vi "Meacurrent8341.vi"(10 "测试类型":u16(ring) items=["DCV", "ACV", "DCI", "ACI", "OHM", "RST", "CAP", "FRQ", "AUTO"], 11 "VISA资源名称":refnum<visa-resource-name>="COM1") -> (0 "错误输出":errorcluster, 2 "数值":dbl format="%#_3g")   [LabVIEW 2013]
uses:
  C:/Program Files/National Instruments/LabVIEW 2013/examples/Instrument IO/Serial/support/Serial - Settings.ctl
  <vilib>/Instr/_visa.llb/VISA Flush IO Buffer Mask.ctl
  <vilib>/Instr/_visa.llb/VISA Configure Serial Port (Instr).vi
panel:
  out "响应":string
  in  "串口设置":T1={"波特率"=9600, "数据比特"=8, "奇偶"=enum."None", "停止位"=10, "流控制"=0} {"流控制" items=["无"=0, "XON/XOFF"=1, "RTS/CTS"=2, "DTR/DSR"=4]; "停止位" items=["1.0"=10, "1.5"=15, "2.0"=20]; "数据比特" min=5 max=8 step=1; "波特率" items=["75"=75, "110"=110, "134"=134, "150"=150, "300"=300, "600"=600, "1200"=1200, "1800"=1800, "2400"=2400, "4800"=4800, "7200"=7200, "9600"=9600, "14400"=14400, "19200"=19200, "28800"=28800, "38400"=38400, "56000"=56000, "57600"=57600, "115200"=115200, "128000"=128000, "230400"=230400]}
  in  "读取前延时(ms)":u32=600
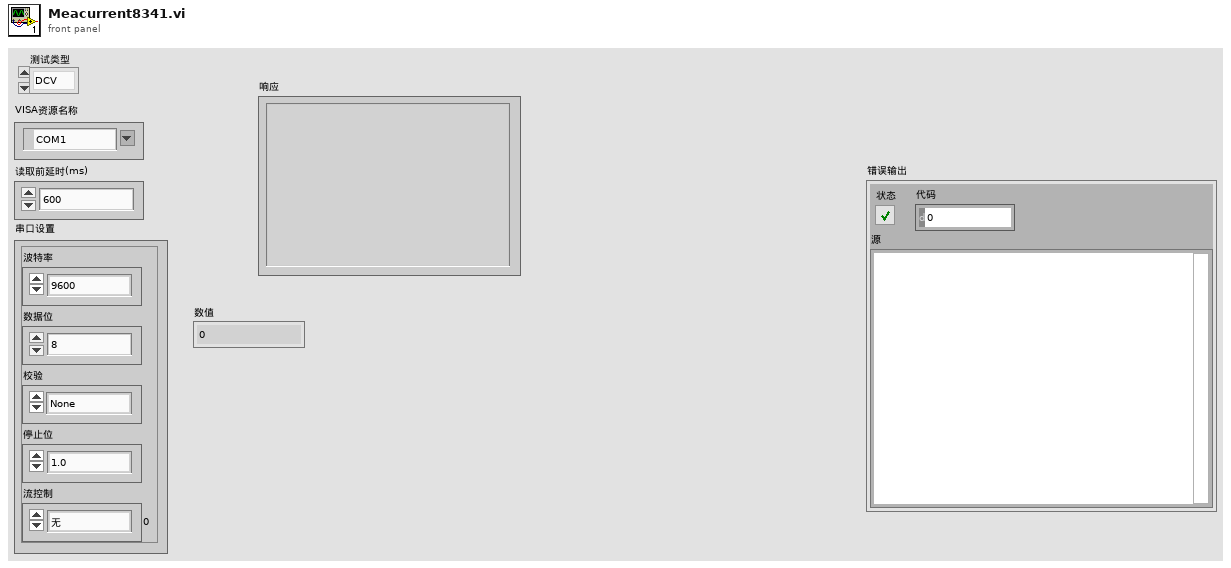
[diagram p1: front panel]
types:
  T1 = typedef "Serial - Settings.ctl" = cluster{"波特率":u32, "数据比特":u16, "奇偶":enum16{"None", "Odd", "Even", "Mark", "Space"}, "停止位":u16, "流控制":u16}
  T2 = typedef "VISA Flush IO Buffer Mask.ctl" = u16
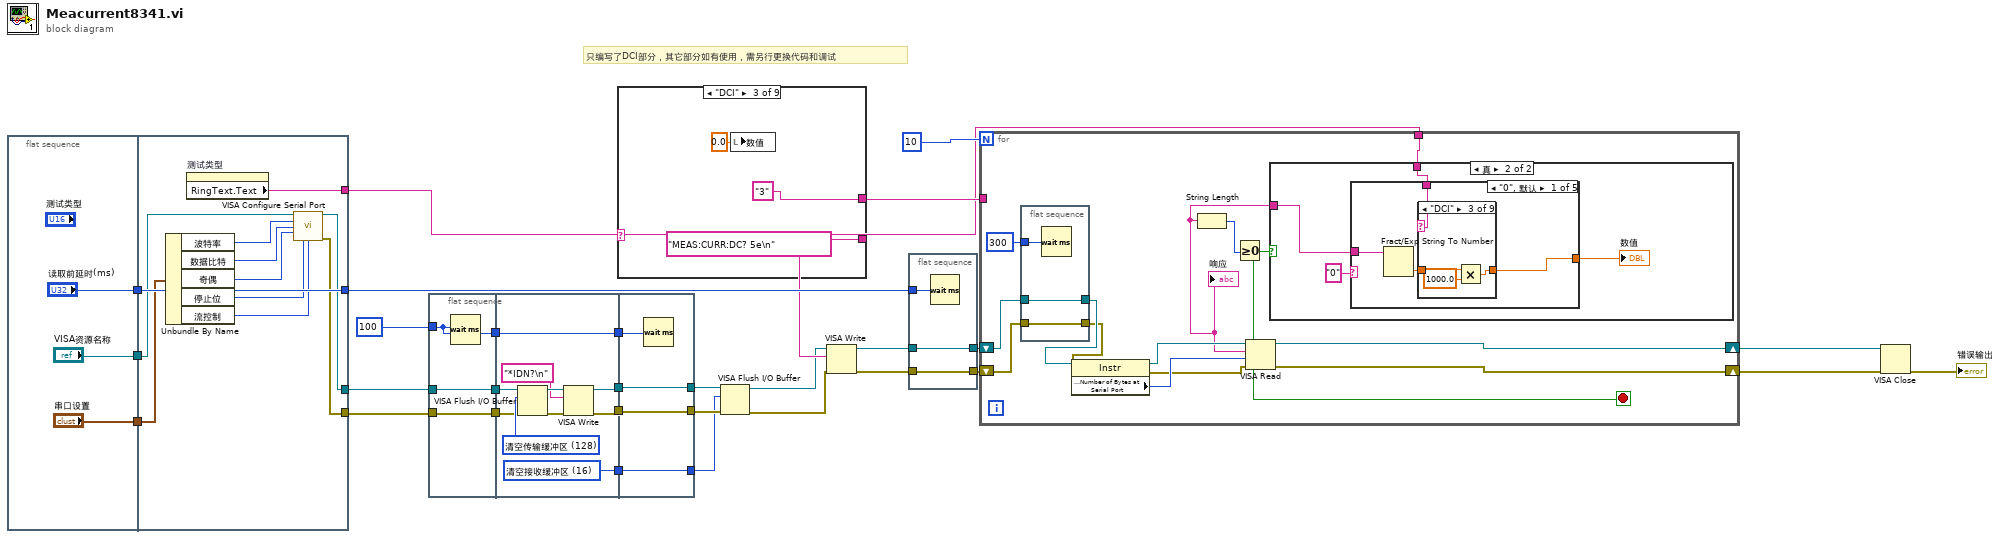
[diagram p0: block diagram]
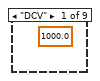
[diagram p3: hidden frame]
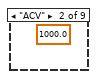
[diagram p4: hidden frame]
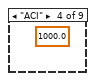
[diagram p5: hidden frame]
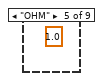
[diagram p6: hidden frame]
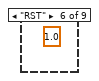
[diagram p7: hidden frame]
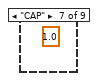
[diagram p8: hidden frame]
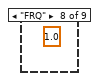
[diagram p9: hidden frame]
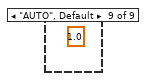
[diagram p10: hidden frame]
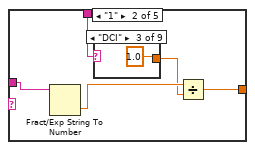
[diagram p11: hidden frame]
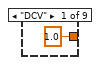
[diagram p12: hidden frame]
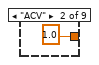
[diagram p13: hidden frame]
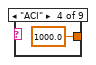
[diagram p14: hidden frame]
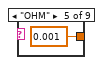
[diagram p15: hidden frame]
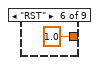
[diagram p16: hidden frame]
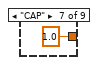
[diagram p17: hidden frame]
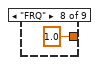
[diagram p18: hidden frame]
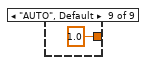
[diagram p19: hidden frame]
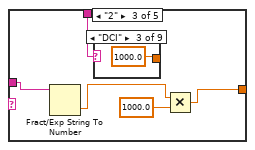
[diagram p20: hidden frame]
diagram:
  # "只编写了DCI部分，其它部分如有使用，需另行更换代码和调试"
  n1 = flat-sequence {
    tunnel: ["VISA资源名称"] -> w8
    tunnel: ["读取前延时(ms)"] -> w7
    tunnel: ["串口设置"] -> w6
    tunnel: [w44] -> w26
    tunnel: w8 -> [w37]
    tunnel: w7 -> [w44]
    tunnel: w6 -> [w38]
    tunnel: [w36] -> w4
    tunnel: [w35] -> w2
    tunnel: [w34] -> w1
    frame #0 {
    }
    frame #1 {
      n2 = Unbundle By Name(w38) -> ("波特率"=w39:u32, "数据比特"=w40:u16, "奇偶"=w41:enum16{"None", "Odd", "Even", "Mark", "Space"}, "停止位"=w42:u16, "流控制"=w43:u16)
      n3 = property on="测试类型" class="Ring (严格)"() -> ("RingText.Text"=w34:string)  [unwired: 2 in, 2 out]
      n4 = call-poly "VISA Configure Serial Port"("VISA resource name"=w37, "baud rate (9600)"=w39, "data bits (8)"=w40, "parity (0:none)"=w41, "stop bits (10: 1 bit)"=w42, "flow control (0:none)"=w43) -> ("VISA resource name out"=w36:refnum<visa-resource-name>, "error out"=w35:errorcluster)  [unwired: 3 in, 5 out]
    }
  }
  n5 = flat-sequence {
    tunnel: u32 100 ("读取前延时(ms)") -> [w47]
    tunnel: [w47] -> w17
    tunnel: [w46] -> w5
    tunnel: w4 -> [w46]
    tunnel: [w45] -> w3
    tunnel: w2 -> [w45]
    tunnel: [w52] -> w20
    tunnel: [w53] -> w19
    tunnel: [w51] -> w18
    tunnel: w17 -> [w51]
    tunnel: [w50] -> w16
    tunnel: w5 -> [w49]
    tunnel: w3 -> [w48]
    tunnel: [w59] -> w13
    tunnel: [w60] -> w12
    tunnel: w20 -> [w60]
    tunnel: w19 -> [w59]
    tunnel: w18 -> [w61]
    tunnel: w16 -> [w58]
    tunnel: [w58] -> w11
    frame #0 {
      n6 = Wait (ms)(milliseconds to wait=w47) -> ()  [unwired: 1 out]
    }
    frame #1 {
      w50 = T2 16 items=["清空接收缓冲区"=16, "向设备写入传输缓冲区"=32, "清空接收缓冲区（无I/O）"=64, "清空传输缓冲区"=128] ("Mask")
      w57 = T2 128 items=["清空接收缓冲区"=16, "向设备写入传输缓冲区"=32, "清空接收缓冲区（无I/O）"=64, "清空传输缓冲区"=128] ("Mask")
      n7 = VISA Flush I/O Buffer(VISA resource name=w49, mask (16)=w57, error in (no error)=w48) -> (VISA resource name out=w55:refnum<visa-resource-name>, error out=w56:errorcluster)
      n8 = VISA Write(VISA resource name=w55, write buffer="*IDN?\n" ("写入缓冲区"), error in (no error)=w56) -> (VISA resource name out=w53:refnum<visa-resource-name>, error out=w52:errorcluster)  [unwired: 1 out]
    }
    frame #2 {
      n9 = Wait (ms)(milliseconds to wait=w61) -> ()  [unwired: 1 out]
    }
  }
  n10 = case shown="\"DCI\"" w1 {
    tunnel: ["AA" ("Command") "BB" ("Command") "MEAS:CURR:DC? 5e\n" "DD" ("Command") "EE" ("Command") "FF" ("Command") "GG" ("Command") "HH" ("Command") "MM" ("Command")] -> w25
    tunnel: ["0" ("Command") "1" ("Command") "3" ("Command") "4" ("Command") "6" ("Command") "F" ("Command") "7" ("Command") "8" ("Command") "M" ("Command")] -> w24
    frame "DCV" {
    }
    frame "ACV" {
    }
    frame "DCI" {
      n11 = local write "数值"(0.0 ("数值")) -> ()
    }
    frame "ACI" {
    }
    frame "OHM" {
    }
    frame "RST" {
    }
    frame "CAP" {
    }
    frame "FRQ" {
    }
    frame "AUTO", Default {
    }
  }
  n12 = VISA Flush I/O Buffer(VISA resource name=w13, mask (16)=w11, error in (no error)=w12) -> (VISA resource name out=w9:refnum<visa-resource-name>, error out=w10:errorcluster)
  n13 = VISA Write(VISA resource name=w9, write buffer=w25, error in (no error)=w10) -> (VISA resource name out=w15:refnum<visa-resource-name>, error out=w14:errorcluster)  [unwired: 1 out]
  n14 = flat-sequence {
    tunnel: [w81] -> w28
    tunnel: [w82] -> w27
    tunnel: w26 -> [w83]
    tunnel: w15 -> [w82]
    tunnel: w14 -> [w81]
    frame #0 {
      n15 = Wait (ms)(milliseconds to wait=w83) -> ()  [unwired: 1 out]
    }
  }
  n16 = for {
    N: 10 -> [_]
    tunnel: w24 -> [_]
    tunnel: w1 -> [w94]
    shift-right: [w96] -> w29
    shift-left: w27 -> [w93]
    shift-right: [w97] -> w30
    shift-left: w28 -> [w91]
    stop <- w88 stop-if-true
    n17 = flat-sequence {
      tunnel: w91 -> [w99]
      tunnel: [w99] -> w90
      tunnel: w93 -> [w98]
      tunnel: [w98] -> w92
      tunnel: u32 300 ("读取前延时(ms)") -> [w100]
      frame #0 {
        n18 = Wait (ms)(milliseconds to wait=w100) -> ()  [unwired: 1 out]
      }
    }
    n19 = property class="Instr"(reference=w92, error in=w90) -> (reference out=w87:refnum<visa-resource-name>, error out=w86:errorcluster, "Serial Settings:Number of Bytes at Serial Port"=w95:u32)
    n20 = VISA Read(VISA resource name=w87, byte count=w95, error in (no error)=w86) -> (VISA resource name out=w96:refnum<visa-resource-name>, read buffer=w84:string, error out=w97:errorcluster)  [unwired: 1 out]
    "响应" <- w84
    n21 = String Length(string=w84) -> (length=w85:i32)
    n22 = Greater Or Equal To 0?(x=w85) -> (x >= 0?=w88:bool)
    n23 = case shown="真" w88 {
      tunnel: w84 -> [_ w101]
      tunnel: w94 -> [_ w104]
      frame False {
      }
      frame True {
        n24 = case shown="\"0\", 默认" "0" {
          tunnel: w101 -> [w108 w116 w130 w144 w158]
          tunnel: w104 -> [w107 w115 w129 w143 w157]
          tunnel: [w106 w112 w126 w140 w154] -> w103
          frame "0", Default {
            n25 = Fract/Exp String To Number(string=w108) -> (number=w105:dbl)  [unwired: 3 in, 1 out]
            n26 = case shown="\"DCI\"" w107 {
              tunnel: [_ _ w109 _ _ _ _ _ _] -> w106
              tunnel: w105 -> [_ _ w111 _ _ _ _ _ _]
              frame "DCV" {
                (unwired) 1000.0
              }
              frame "ACV" {
                (unwired) 1000.0
              }
              frame "DCI" {
                n27 = Multiply(x=w111, y=1000.0) -> (x*y=w109:dbl)
              }
              frame "ACI" {
                (unwired) 1000.0
              }
              frame "OHM" {
                (unwired) 1.0
              }
              frame "RST" {
                (unwired) 1.0
              }
              frame "CAP" {
                (unwired) 1.0
              }
              frame "FRQ" {
                (unwired) 1.0
              }
              frame "AUTO", Default {
                (unwired) 1.0
              }
            }
          }
          frame "1" {
            n28 = Fract/Exp String To Number(string=w116) -> (number=w114:dbl)  [unwired: 3 in, 1 out]
            n29 = case shown="\"DCI\"" w115 {
              tunnel: [1.0 1.0 1.0 1000.0 0.001 1.0 1.0 1.0 1.0] -> w113
              frame "DCV" {
              }
              frame "ACV" {
              }
              frame "DCI" {
              }
              frame "ACI" {
              }
              frame "OHM" {
              }
              frame "RST" {
              }
              frame "CAP" {
              }
              frame "FRQ" {
              }
              frame "AUTO", Default {
              }
            }
            n30 = Divide(x=w114, y=w113) -> (x/y=w112:dbl)
          }
          frame "2" {
            n31 = Fract/Exp String To Number(string=w130) -> (number=w128:dbl)  [unwired: 3 in, 1 out]
            n32 = case shown="\"DCI\"" w129 {
              tunnel: [1.0 1.0 1000.0 1000.0 0.001 1.0 1.0 1.0 1.0] -> _
              frame "DCV" {
              }
              frame "ACV" {
              }
              frame "DCI" {
              }
              frame "ACI" {
              }
              frame "OHM" {
              }
              frame "RST" {
              }
              frame "CAP" {
              }
              frame "FRQ" {
              }
              frame "AUTO", Default {
              }
            }
            n33 = Multiply(x=w128, y=1000.0) -> (x*y=w126:dbl)
          }
          frame "3" {
            n34 = Fract/Exp String To Number(string=w144) -> (number=w142:dbl)  [unwired: 3 in, 1 out]
            n35 = case shown="\"DCI\"" w143 {
              tunnel: [1.0 1.0 1000.0 1000.0 0.001 1.0 1.0 1.0 1.0] -> w141
              frame "DCV" {
              }
              frame "ACV" {
              }
              frame "DCI" {
              }
              frame "ACI" {
              }
              frame "OHM" {
              }
              frame "RST" {
              }
              frame "CAP" {
              }
              frame "FRQ" {
              }
              frame "AUTO", Default {
              }
            }
            n36 = Divide(x=w142, y=w141) -> (x/y=w140:dbl)
          }
          frame "4" {
            n37 = Fract/Exp String To Number(string=w158) -> (number=w156:dbl)  [unwired: 3 in, 1 out]
            n38 = case shown="\"DCI\"" w157 {
              tunnel: [1.0 1.0 1000.0 1000.0 1e-06 1.0 1.0 1.0 1.0] -> w155
              frame "DCV" {
              }
              frame "ACV" {
              }
              frame "DCI" {
              }
              frame "ACI" {
              }
              frame "OHM" {
              }
              frame "RST" {
              }
              frame "CAP" {
              }
              frame "FRQ" {
              }
              frame "AUTO", Default {
              }
            }
            n39 = Divide(x=w156, y=w155) -> (x/y=w154:dbl)
          }
        }
        "数值" <- w103
      }
    }
  }
  n40 = VISA Close(VISA resource name=w29, error in (no error)=w30) -> (error out=→"错误输出":errorcluster)
